vi "test core.vi"(8 "error in (no error)":errorcluster, 11 "File Actor in":refnum<class "File Actor.lvclass">) -> (0 "error out":errorcluster)   [LabVIEW 2014, in "File Library.lvlib" / "File Actor.lvclass"]
uses:
  File Actor.lvclass
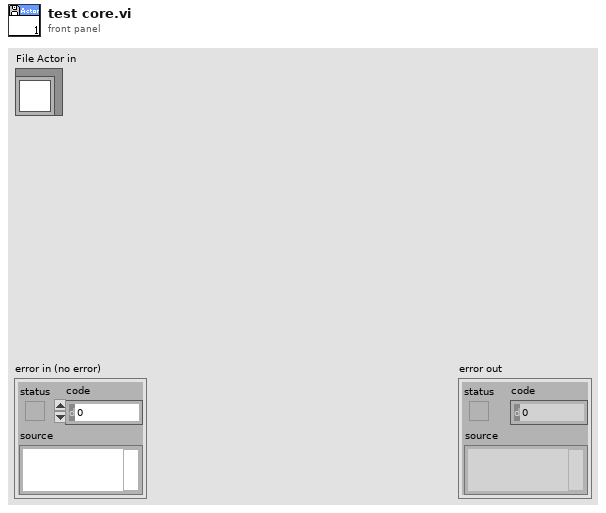
[diagram p1: front panel]
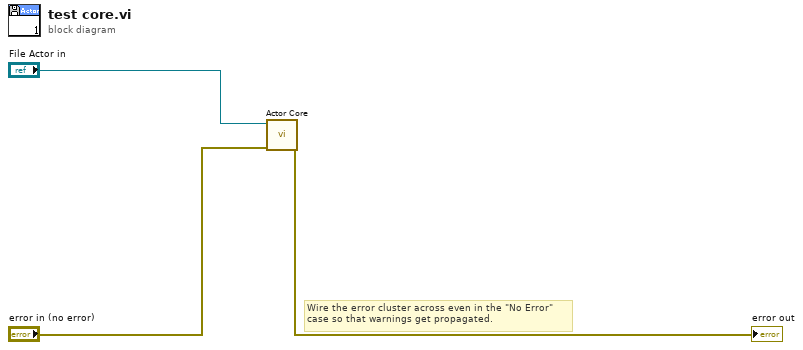
[diagram p0: block diagram]
diagram:
  # "Wire the error cluster across even in the \"No Error\"\ncase so that warnings get propagated."
  n1 = call-dynamic "Actor Core.vi"("error in"="error in (no error)", "File Actor in"="File Actor in") -> ("error out"=→"error out":errorcluster)  [unwired: 8 in, 1 out]
